vi "Set Delay Method.vi"   [LabVIEW 2016, in "Delay Line.lvlib" / "Abstract Delay Line.lvclass"]
uses:
  Abstract Delay Line.lvclass
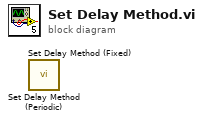
[diagram p0: block diagram]
diagram:
  n1 = call-dynamic "Set Delay Method (Periodic).vi"() -> ()  [unwired: 10 in, 2 out]
  n2 = call-dynamic "Set Delay Method (Fixed).vi"() -> ()  [unwired: 10 in, 2 out]
